vi "DataToCSV.vi"(4 "MagnetometerZ":dbl, 5 "Arreter":bool, 6 "MagnetometerY":dbl, 7 "Delai en ms":dbl, 8 "MagnetometerX":dbl, 9 "AccelometerZ":dbl, 10 "AccelometerY":dbl, 11 "AccelometerX":dbl format="%#_6f") -> ()   [LabVIEW 2019]
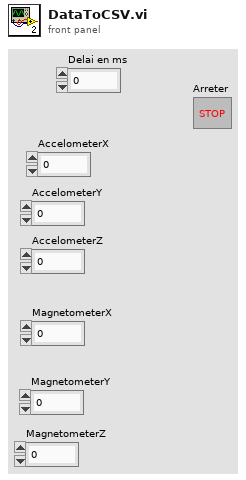
[diagram p1: front panel]
types:
  T1 = enum16{"open", "replace", "create", "open or create", "replace or create", "replace or create with confirmation"}
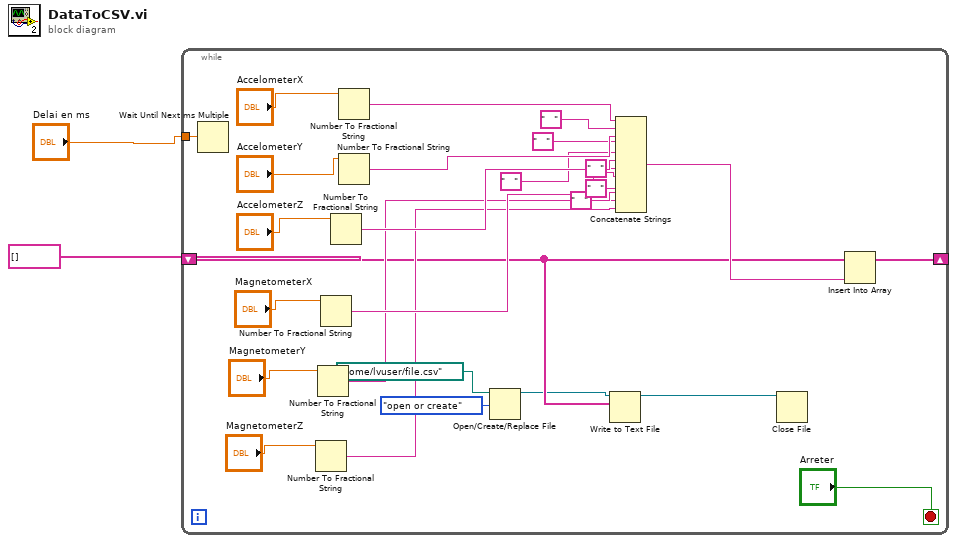
[diagram p0: block diagram]
diagram:
  n1 = while {
    shift-right: [w29] -> _
    shift-left: string[] [] -> [w9]
    tunnel: "Delai en ms" -> [w3]
    stop <- "Arreter" stop-if-true
    n2 = Wait Until Next ms Multiple(millisecond multiple=w3) -> ()  [unwired: 1 out]
    n3 = Number To Fractional String(number="MagnetometerZ") -> (F-format string=w17:string)  [unwired: 3 in]
    n4 = Number To Fractional String(number="MagnetometerY") -> (F-format string=w18:string)  [unwired: 3 in]
    n5 = Number To Fractional String(number="MagnetometerX") -> (F-format string=w19:string)  [unwired: 3 in]
    n6 = Number To Fractional String(number="AccelometerZ") -> (F-format string=w20:string)  [unwired: 3 in]
    n7 = Number To Fractional String(number="AccelometerX") -> (F-format string=w22:string)  [unwired: 3 in]
    n8 = Number To Fractional String(number="AccelometerY") -> (F-format string=w21:string)  [unwired: 3 in]
    n9 = Open/Create/Replace File(file path (use dialog)=path "/home/lvuser/file.csv", operation (0:open)=T1."open or create") -> (refnum out=w6:refnum<file>)  [unwired: 4 in, 2 out]
    n10 = Write to Text File(file (use dialog)=w6, text=w9) -> (refnum out=w5:refnum<file>)  [unwired: 2 in, 2 out]
    n11 = Concatenate Strings(w22, "   " ("string"), w21, "   " ("string"), "   " ("string"), w20, "   " ("string"), w19, "   " ("string"), w18, "   " ("string"), w17) -> (w10:string)
    n12 = Close File(refnum=w5) -> ()  [unwired: 1 in, 2 out]
    n13 = Insert Into Array(array=w9, new element=w10) -> (w29:string[])  [unwired: 1 in]
  }
